vi "testNewDBConnection.vi"() -> ()   [LabVIEW 2009, in "run.lvlib"]
uses:
  run.lvlib
  Tools/DatabaseHelpers/DbConnection/DeviceDataBase/deviceDataBase.lvclass
  Tools/DatabaseHelpers/Database Objects/ChannelArray/ChannelArray.lvclass
  Tools/DatabaseHelpers/Database Objects/Channel/Channel.lvclass
  Tools/DatabaseHelpers/Database Objects/DeviceArray/DeviceArray.lvclass
  Tools/DatabaseHelpers/Database Objects/device/device.lvclass
panel:
  out "total":dbl format="%_9g"
  out "channelNames":string[](array[string])
  out "size(s)":i32
  out "safestates":T1(array[cluster])=[{"Frequency(MHz)"=100.0, "Amplitude"=1.0, "Phase"=0.0, "OutputForm"=enum."Sine"}, {"Frequency(MHz)"=100.0, "Amplitude"=1.0, "Phase"=0.0, "OutputForm"=enum."Sine"}]
  out "ChannelAddresses":string[](array[string])
  out "channels_inUse":T2(array[cluster])
  out "triggering":T3(array[cluster])
  out "devices":string[](array[string])
  out "state":cluster{"type":string, "channel_name":string}[](array[cluster])
  out "channels":string[](array[string])
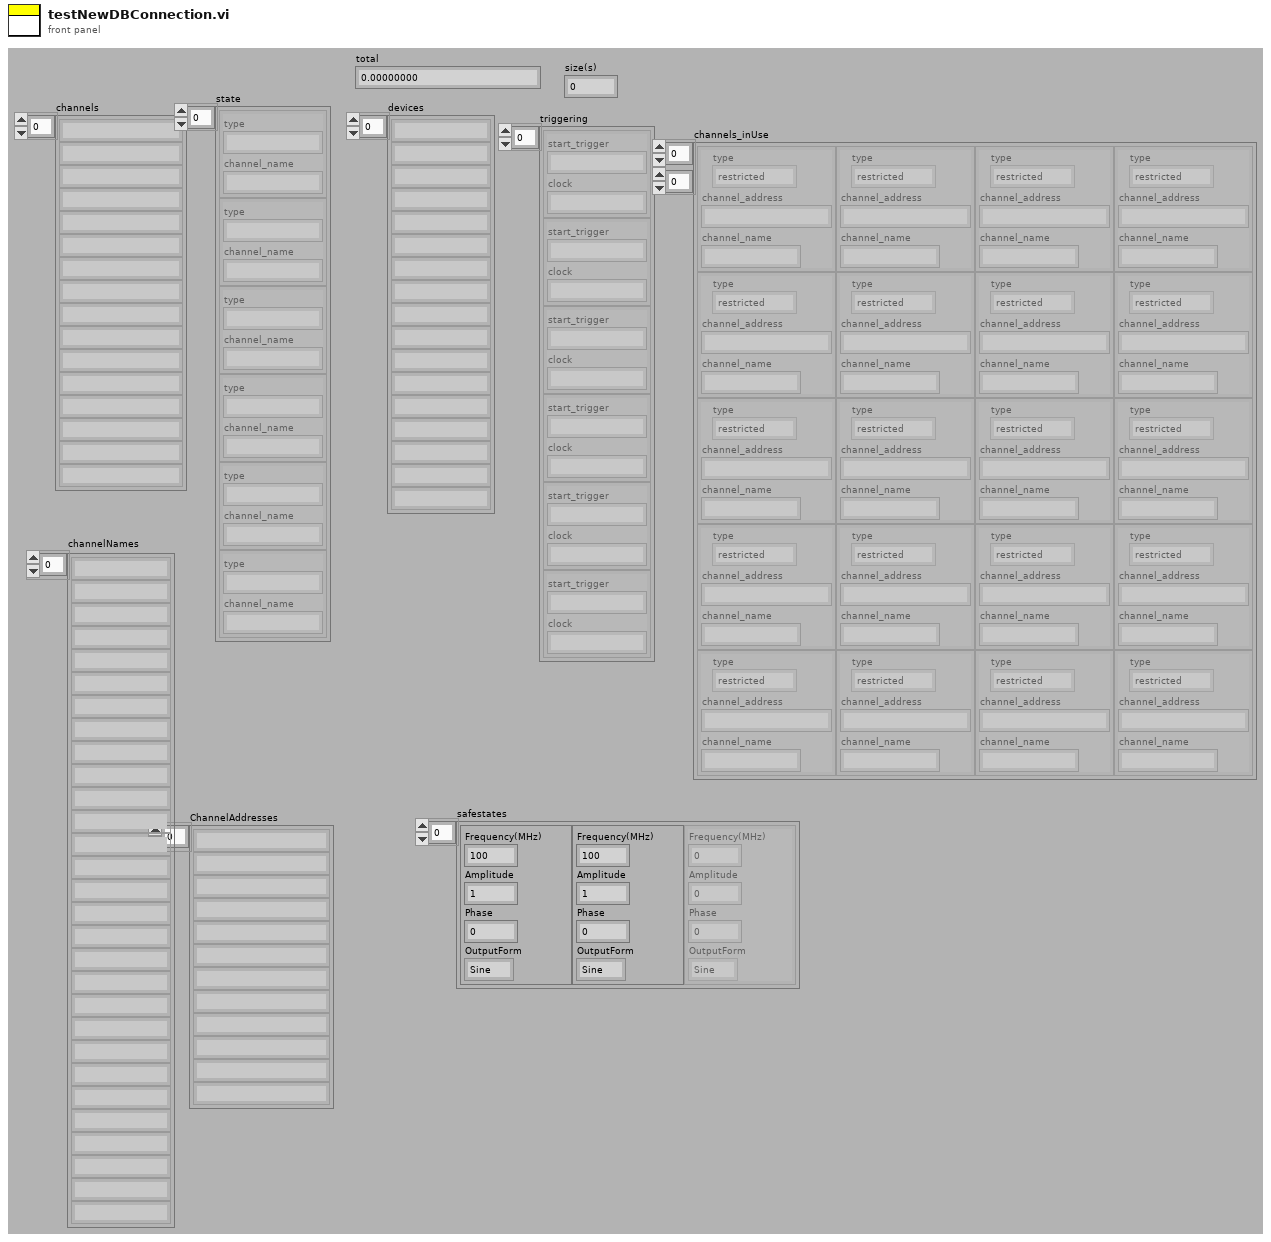
[diagram p1: front panel]
types:
  T1 = cluster{"Frequency(MHz)":dbl, "Amplitude":dbl, "Phase":dbl, "OutputForm":enum16{"Sine", "Square", "Triangle", "Arbitrary"}}[]
  T2 = cluster{"type":enum16{"restricted", "unrestricted"}, "channel_address":string, "channel_name":string}[][]
  T3 = cluster{"start_trigger":string, "clock":string}[]
  T4 = cluster{"type":enum16{"restricted", "unrestricted"}, "channel_address":string, "channel_name":string}[]
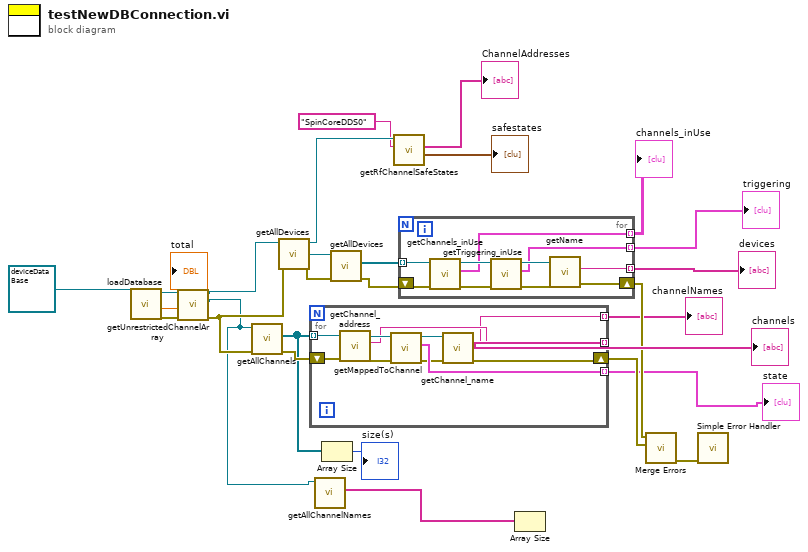
[diagram p0: block diagram]
diagram:
  n1 = call "loadDatabase.vi"("deviceDataBase in"=refnum<class "deviceDataBase.lvclass"> refnum) -> ("error out"=w14:errorcluster, "total"=→"total":dbl, "deviceDataBase out"=w16:refnum<class "deviceDataBase.lvclass">)  [unwired: 8 in]
  n2 = call "getUnrestrictedChannelArray.vi"("error in (no error)"=w14, "deviceDataBase in"=w16) -> ("error out"=w13:errorcluster, "ChannelArray.lvclass"=w4:refnum<class "ChannelArray.lvclass">, "deviceDataBase out"=w15:refnum<class "deviceDataBase.lvclass">)  [unwired: 7 in]
  n3 = call "getAllChannels.vi"("error in (no error)"=w13, "ChannelArray.lvclass in"=w4) -> ("error out"=w26:errorcluster, "channels"=w6:refnum<class "Channel.lvclass">[])  [unwired: 7 in, 1 out]
  n4 = call "getAllDevices.vi"("error in (no error)"=w13, "deviceDataBase in"=w15) -> ("error out"=w8:errorcluster, "deviceArray.lvclass"=w25:refnum<class "DeviceArray.lvclass">, "deviceDataBase out"=w12:refnum<class "deviceDataBase.lvclass">)  [unwired: 7 in]
  n5 = for {
    tunnel: w6 -> [w37] mode=indexing
    tunnel: [w33] -> w27 mode=indexing
    shift-right: [w31] -> w18
    shift-left: w26 -> [w36]
    tunnel: [w32] -> w7 mode=indexing
    tunnel: [w29] -> w2 mode=indexing
    n6 = call "getChannel_address.vi"("error in (no error)"=w36, "Channel.lvclass in"=w37) -> ("error out"=w35:errorcluster, "channel_address"=w33:string, "Channel.lvclass out"=w34:refnum<class "Channel.lvclass">)  [unwired: 7 in]
    n7 = call "getMappedToChannel.vi"("error in (no error)"=w35, "Channel.lvclass in"=w34) -> ("error out"=w31:errorcluster, "mappedTo"=w32:cluster{"type":string, "channel_name":string}, "Channel.lvclass out"=w30:refnum<class "Channel.lvclass">)  [unwired: 7 in]
    n8 = call "getChannel_name.vi"("Channel.lvclass in"=w30) -> ("channel_name"=w29:string)  [unwired: 8 in, 2 out]
  }
  "channels" <- w27
  "state" <- w7
  "channelNames" <- w2
  n9 = call "getAllChannelNames.vi"("ChannelArray in"=w4) -> ("channelNames"=w3:string[])  [unwired: 8 in, 2 out]
  n10 = Array Size(array=w6) -> (size(s)=→"size(s)":i32)
  n11 = call "getAllDevices.vi"("error in (no error)"=w8, "DeviceArray.lvclass in"=w25) -> ("error out"=w24:errorcluster, "deviceArray"=w23:refnum<class "device.lvclass">[])  [unwired: 7 in, 1 out]
  n12 = call "getRfChannelSafeStates.vi"("deviceName"="SpinCoreDDS0", "deviceDataBase in"=w12) -> ("safestates"=→"safestates":T1, "ChannelAddresses"=→"ChannelAddresses":string[])  [unwired: 6 in, 2 out]
  n13 = for {
    shift-right: [w38] -> w19
    shift-left: w24 -> [w47]
    tunnel: w23 -> [w46] mode=indexing
    tunnel: [w41] -> w20 mode=indexing
    tunnel: [w40] -> w21 mode=indexing
    tunnel: [w39] -> w22 mode=indexing
    n14 = call "getChannels_inUse.vi"("error in (no error)"=w47, "device.lvclass in"=w46) -> ("error out"=w44:errorcluster, "channels_inUse"=w41:T4, "device.lvclass out"=w43:refnum<class "device.lvclass">)  [unwired: 7 in]
    n15 = call "getTriggering_inUse.vi"("error in (no error)"=w44, "device.lvclass in"=w43) -> ("error out"=w45:errorcluster, "triggering_inUse"=w40:cluster{"start_trigger":string, "clock":string}, "device.lvclass out"=w42:refnum<class "device.lvclass">)  [unwired: 7 in]
    n16 = call "getName.vi"("error in (no error)"=w45, "device.lvclass in"=w42) -> ("error out"=w38:errorcluster, "name"=w39:string)  [unwired: 7 in, 1 out]
  }
  "devices" <- w22
  "triggering" <- w21
  "channels_inUse" <- w20
  n17 = Array Size(array=w3) -> ()  [unwired: 1 out]
  n18 = call <vilib>:"Merge Errors.vi"("error in 2 (no error)"=w18, "error in 1 (no error)"=w19) -> ("error out"=w17:errorcluster)  [unwired: 5 in]
  n19 = call <vilib>:"Simple Error Handler.vi"("error in (no error)"=w17) -> ()  [unwired: 4 in, 5 out]
